vi "Get Bus Controller and Remote Terminals Handles from BTI Channel.vi"(8 "error in":errorcluster, 11 "channel handle in":u64) -> (0 "error out":errorcluster, 1 "remote terminal handles out":u64[](array[numeric]), 2 "bus controller handle out":u64, 3 "channel handle out":u64)   [LabVIEW 2020, in "Ballard MIL-STD-1553 Engine.lvlib" / "Custom Device.lvlib"]
uses:
  Custom Device.lvlib
  <instrlib>/BTI1553Lib/BTI1553LV.lvlib
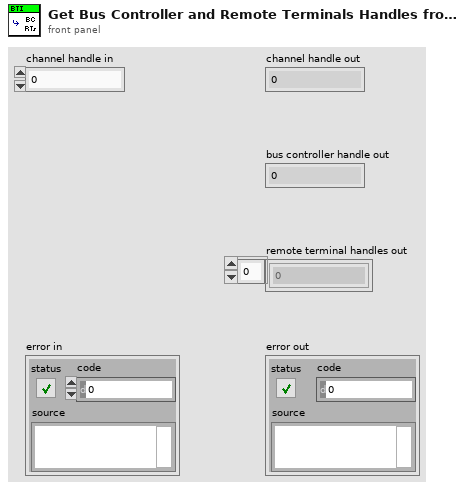
[diagram p1: front panel]
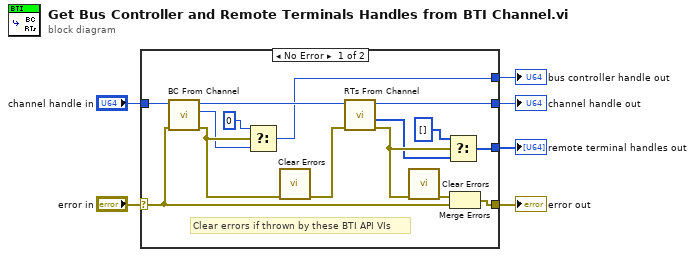
[diagram p0: block diagram]
diagram:
  n1 = case shown="No Error" "error in" {
    selector: "error in" -> [w8 w22]
    tunnel: [w14 _] -> w6
    tunnel: "channel handle in" -> [w20 w23]
    tunnel: [w10 _] -> w3
    tunnel: [w7 w22] -> w2
    tunnel: [w19 w23] -> w1
    frame No Error {
      # "Clear errors if thrown by these BTI API VIs"
      n2 = call <instrlib>:"BC From Channel.vi"("error in (no error)"=w8, "channel handle in"=w20) -> ("error out"=w17:errorcluster, "bus controller handle out"=w16:u64, "channel handle out"=w21:u64)  [unwired: 7 in]
      n3 = Select(t=u64 0, s=w17, f=w16) -> (s? t:f=w14:u64)
      n4 = call <vilib>:"Clear Errors.vi"("error in (no error)"=w17) -> ("error out"=w18:errorcluster)  [unwired: 5 in, 1 out]
      n5 = call <instrlib>:"RTs From Channel.vi"("error in (no error)"=w18, "channel handle in"=w21) -> ("error out"=w13:errorcluster, "remote terminal handles out"=w12:u64[], "channel handle out"=w19:u64)  [unwired: 6 in, 1 out]
      n6 = call <vilib>:"Clear Errors.vi"("error in (no error)"=w13) -> ("error out"=w9:errorcluster)  [unwired: 5 in, 1 out]
      n7 = Select(t=u64[] [], s=w13, f=w12) -> (s? t:f=w10:u64[])
      n8 = Merge Errors(w9, w8) -> (w7:errorcluster)
    }
    frame Error {
    }
  }
  "bus controller handle out" <- w6
  "remote terminal handles out" <- w3
  "error out" <- w2
  "channel handle out" <- w1
